vi "Write External Network Present.vi"(8 "error in (no error)":errorcluster, 10 "External Network Present":bool, 11 "QPA Measurement in":refnum<class "QPA Measurement.lvclass">=refnum) -> (0 "error out":errorcluster, 3 "QPA Measurement out":refnum<class "QPA Measurement.lvclass">)   [LabVIEW 2016, in "QPA Measurement.lvlib" / "QPA Measurement.lvclass"]
uses:
  QPA Measurement.lvclass
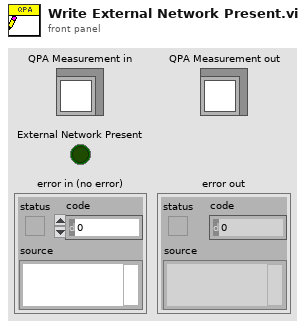
[diagram p1: front panel]
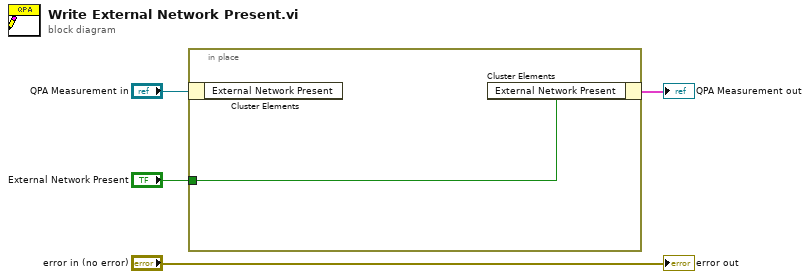
[diagram p0: block diagram]
diagram:
  n1 = in-place {
    in-place-border: "External Network Present" -> [w5]
    n2 = in-place-cluster #1("QPA Measurement in") -> ()  [unwired: 1 out]
    n3 = in-place-cluster #1("External Network Present"=w5) -> (→"QPA Measurement out":cluster{})
  }
  "error out" <- "error in (no error)"
